vi "_Configure Window.vi"(4 "For Printing (T)":bool=TRUE, 6 "Expt#":i32=1, 7 "ControlRef":T1) -> ()   [LabVIEW 2012]
uses:
  Type/_Run Module.ctl
  Type/_Data Operation.ctl
  Configuration/_Global Configuration.vi
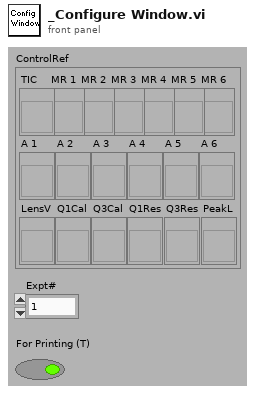
[diagram p1: front panel]
types:
  T1 = cluster{"TIC":refnum<vi>, "MR 1":refnum<vi>, "MR 2":refnum<vi>, "MR 3":refnum<vi>, "MR 4":refnum<vi>, "MR 5":refnum<vi>, "MR 6":refnum<vi>, "A 1":refnum<vi>, "A 2":refnum<vi>, "A 3":refnum<vi>, "A 4":refnum<vi>, "A 5":refnum<vi>, "A 6":refnum<vi>, "LensV":refnum<vi>, "Q1Cal":refnum<vi>, "Q3Cal":refnum<vi>, "Q1Res":refnum<vi>, "Q3Res":refnum<vi>, "PeakL":refnum<vi>}
  T2 = typedef "_Run Module.ctl" = u16
  T3 = typedef "_Data Operation.ctl" = enum8{"Initialize", "Get Data", "Set Data", "Close"}
  T4 = typedef "_Lens Property.ctl" = cluster{"Scan Type":u8, "Scans":i32, "Time 1":dbl, "Time 2":dbl, "Value 1":dbl, "Value 2":dbl, "Step Size":dbl}
  T5 = typedef "_Mass Range Property.ctl" = cluster{"Start":dbl, "Stop":dbl, "Step Size":dbl, "Steps":i32, "Dwell":dbl, "Parameters":T6[], "Res":T7}
  T6 = typedef "_Mass Range Parameters.ctl" = cluster{"Name":string, "Ch#":u8, "StartV":dbl, "StopV":dbl, "StepV":dbl, "Index":u8}
  T7 = typedef "_RT Res Type.ctl" = u16
  T8 = typedef "_Run Mode.ctl" = enum16{"MRM (Q1/Q2)", "Q1 Scan", "Q1 SRM", "Q2 Scan", "Q2 SRM", "Product Scan", "Precursor Scan", "Neutral Loss", "Neutral Gain"}
  T9 = cluster{"Lenses":T4[], "Mass Ranges":T5[], "Acquire":bool, "MCA":bool, "Q1DC EN":bool, "Q1 POL":bool, "Q3 POL":bool, "Q1 RF  EN":bool, "Averaging":bool, "Log Scale":bool, "CPS":bool, "Unit":bool, "Data Path":path, "Run Mode":T8, "Fixed Mass (amu)":dbl, "Q3DC EN":bool, "Q3 RF  EN":bool, "Negative":bool}
  T10 = typedef "_Current Data.ctl" = cluster{"Scan#":i32, "Run Time (mS)":i32, "TIC X":dbl[], "TIC Y":dbl[][], "MassRange":cluster{"X Title":string, "X":dbl[], "Y":i32[]}[], "Fixed Mass (amu)":dbl, "Method":T11}
  T11 = typedef "_XML Expt.ctl" = cluster{"StartT(mS)":i32, "#Cycles":i32, "PauseT(uS)":i32, "ScanType":i32, "Polarity":u8, "FixedMass":dbl, "DelayT(mS)":i32, "Active Ch":T12[], "Mass Range":T5[]}
  T12 = typedef "_XML Lens.ctl" = cluster{"Value":dbl, "ChID":u8}
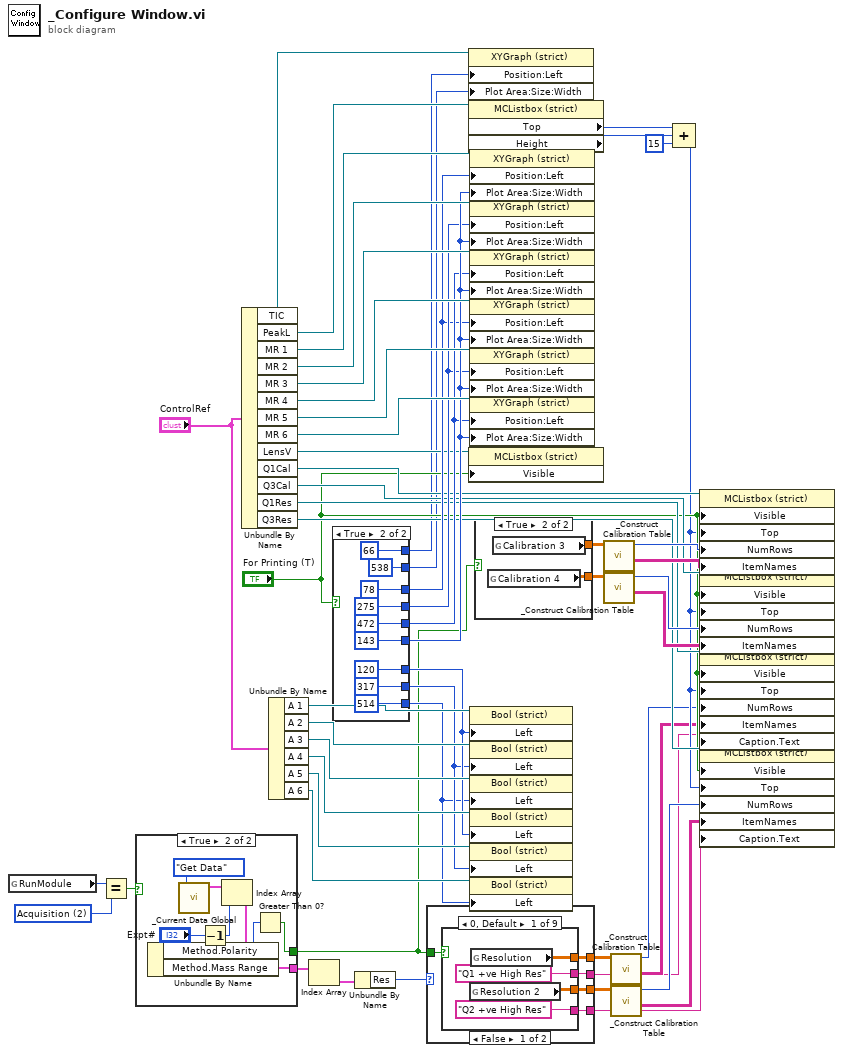
[diagram p0: block diagram]
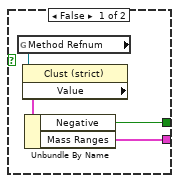
[diagram p2: hidden frame]
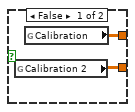
[diagram p3: hidden frame]
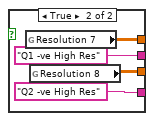
[diagram p4: hidden frame]
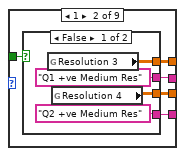
[diagram p5: hidden frame]
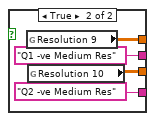
[diagram p6: hidden frame]
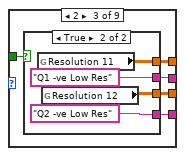
[diagram p7: hidden frame]
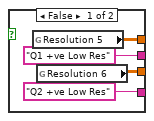
[diagram p8: hidden frame]
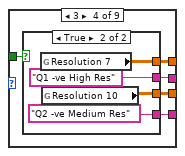
[diagram p9: hidden frame]
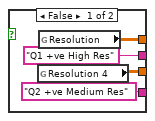
[diagram p10: hidden frame]
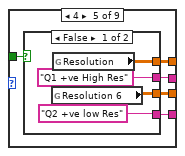
[diagram p11: hidden frame]
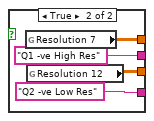
[diagram p12: hidden frame]
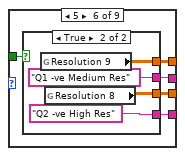
[diagram p13: hidden frame]
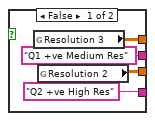
[diagram p14: hidden frame]
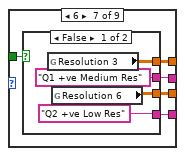
[diagram p15: hidden frame]
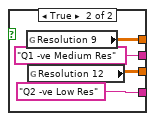
[diagram p16: hidden frame]
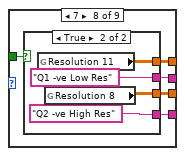
[diagram p17: hidden frame]
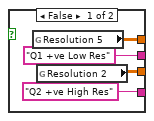
[diagram p18: hidden frame]
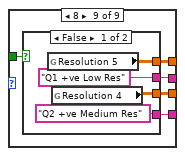
[diagram p19: hidden frame]
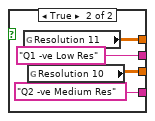
[diagram p20: hidden frame]
diagram:
  w6 = T2 2 items=["Diagnostics", "Tune", "Acquisition"] ("y")
  n1 = global read "_Global Configuration.vi" "RunModule"() -> (w7:T2)
  n2 = Equal?(x=w7, y=w6) -> (x = y?=w5:bool)
  n3 = case shown="True" w5 {
    tunnel: [w57 w63] -> w15
    tunnel: [w56 w62] -> w8
    frame False {
      n4 = global read "_Global Configuration.vi" "Method Refnum"() -> (w59:refnum<vi>)
      n5 = property class="Clust (strict)"(reference=w59) -> ("Value"=w58:T9)  [unwired: 1 in, 2 out]
      n6 = Unbundle By Name(w58) -> ("Negative"=w56:bool, "Mass Ranges"=w57:T5[])
    }
    frame True {
      n7 = call "_Current Data Global.vi"("Operation"=_Data_Operation."Get Data") -> ("CurrentData"=w66:T10[])  [unwired: 3 in, 3 out]
      n8 = Decrement(x="Expt#") -> (x-1=w60:i32)
      n9 = Index Array(array=w66, index=w60) -> (element=w64:T10)
      n10 = Unbundle By Name(w64) -> ("Method.Polarity"=w61:u8, "Method.Mass Range"=w63:T5[])
      n11 = Greater Than 0?(x=w61) -> (x > 0?=w62:bool)
    }
  }
  n12 = Unbundle By Name("ControlRef") -> ("TIC"=w3:refnum<vi>, "PeakL"=w35:refnum<vi>, "MR 1"=w55:refnum<vi>, "MR 2"=w53:refnum<vi>, "MR 3"=w52:refnum<vi>, "MR 4"=w51:refnum<vi>, "MR 5"=w50:refnum<vi>, "MR 6"=w54:refnum<vi>, "LensV"=w45:refnum<vi>, "Q1Cal"=w34:refnum<vi>, "Q3Cal"=w27:refnum<vi>, "Q1Res"=w23:refnum<vi>, "Q3Res"=w22:refnum<vi>)
  n13 = Unbundle By Name("ControlRef") -> ("A 1"=w44:refnum<vi>, "A 2"=w43:refnum<vi>, "A 3"=w42:refnum<vi>, "A 4"=w41:refnum<vi>, "A 5"=w40:refnum<vi>, "A 6"=w39:refnum<vi>)
  n14 = Index Array(array=w15) -> (element=w14:T5)  [unwired: 1 in]
  n15 = case shown="True" "For Printing (T)" {
    tunnel: [-52 ("Position:Left") 78 ("Position:Left")] -> w46
    tunnel: [189 ("Plot Area:Size:Width") 275 ("Plot Area:Size:Width")] -> w47
    tunnel: [429 ("Plot Area:Size:Width") 472 ("Plot Area:Size:Width")] -> w48
    tunnel: [u32 186 ("Plot Area:Size:Width") u32 143 ("Plot Area:Size:Width")] -> w49
    tunnel: [-10 ("Position:Left") 120 ("Position:Left")] -> w38
    tunnel: [231 ("Plot Area:Size:Width") 317 ("Plot Area:Size:Width")] -> w37
    tunnel: [471 ("Plot Area:Size:Width") 514 ("Plot Area:Size:Width")] -> w36
    tunnel: [-64 ("Position:Left") 66 ("Position:Left")] -> w2
    tunnel: [u32 668 ("Plot Area:Size:Width") u32 538 ("Plot Area:Size:Width")] -> w1
    frame False {
    }
    frame True {
    }
  }
  n16 = Unbundle By Name(w14) -> ("Res"=w13:T7)
  n17 = case shown="0, Default" w13 {
    tunnel: [w90 w103 w116 w129 w142 w155 w168 w181 w194] -> w12
    tunnel: [w89 w102 w115 w128 w141 w154 w167 w180 w193] -> w11
    tunnel: [w88 w101 w114 w127 w140 w153 w166 w179 w192] -> w10
    tunnel: [w87 w100 w113 w126 w139 w152 w165 w178 w191] -> w9
    tunnel: w8 -> [w86 w99 w112 w125 w138 w151 w164 w177 w190]
    frame 0, Default {
      n18 = case shown="False" w86 {
        tunnel: [w94 w98] -> w90
        tunnel: [w93 w96] -> w89
        tunnel: ["Q1 +ve High Res" "Q1 -ve High Res"] -> w88
        tunnel: ["Q2 +ve High Res" "Q2 -ve High Res"] -> w87
        frame False {
          n19 = global read "_Global Configuration.vi" "Resolution 2"() -> (w93:dbl[][])
          n20 = global read "_Global Configuration.vi" "Resolution"() -> (w94:dbl[][])
        }
        frame True {
          n21 = global read "_Global Configuration.vi" "Resolution 7"() -> (w98:dbl[][])
          n22 = global read "_Global Configuration.vi" "Resolution 8"() -> (w96:dbl[][])
        }
      }
    }
    frame 1 {
      n23 = case shown="False" w99 {
        tunnel: [w107 w111] -> w103
        tunnel: [w106 w109] -> w102
        tunnel: ["Q1 +ve Medium Res" "Q1 -ve Medium Res"] -> w101
        tunnel: ["Q2 +ve Medium Res" "Q2 -ve Medium Res"] -> w100
        frame False {
          n24 = global read "_Global Configuration.vi" "Resolution 3"() -> (w107:dbl[][])
          n25 = global read "_Global Configuration.vi" "Resolution 4"() -> (w106:dbl[][])
        }
        frame True {
          n26 = global read "_Global Configuration.vi" "Resolution 9"() -> (w111:dbl[][])
          n27 = global read "_Global Configuration.vi" "Resolution 10"() -> (w109:dbl[][])
        }
      }
    }
    frame 2 {
      n28 = case shown="True" w112 {
        tunnel: [w120 w124] -> w116
        tunnel: [w119 w122] -> w115
        tunnel: ["Q1 +ve Low Res" "Q1 -ve Low Res"] -> w114
        tunnel: ["Q2 +ve Low Res" "Q2 -ve Low Res"] -> w113
        frame False {
          n29 = global read "_Global Configuration.vi" "Resolution 5"() -> (w120:dbl[][])
          n30 = global read "_Global Configuration.vi" "Resolution 6"() -> (w119:dbl[][])
        }
        frame True {
          n31 = global read "_Global Configuration.vi" "Resolution 11"() -> (w124:dbl[][])
          n32 = global read "_Global Configuration.vi" "Resolution 12"() -> (w122:dbl[][])
        }
      }
    }
    frame 3 {
      n33 = case shown="True" w125 {
        tunnel: [w133 w137] -> w129
        tunnel: [w132 w135] -> w128
        tunnel: ["Q1 +ve High Res" "Q1 -ve High Res"] -> w127
        tunnel: ["Q2 +ve Medium Res" "Q2 -ve Medium Res"] -> w126
        frame False {
          n34 = global read "_Global Configuration.vi" "Resolution 4"() -> (w132:dbl[][])
          n35 = global read "_Global Configuration.vi" "Resolution"() -> (w133:dbl[][])
        }
        frame True {
          n36 = global read "_Global Configuration.vi" "Resolution 7"() -> (w137:dbl[][])
          n37 = global read "_Global Configuration.vi" "Resolution 10"() -> (w135:dbl[][])
        }
      }
    }
    frame 4 {
      n38 = case shown="False" w138 {
        tunnel: [w146 w150] -> w142
        tunnel: [w145 w148] -> w141
        tunnel: ["Q1 +ve High Res" "Q1 -ve High Res"] -> w140
        tunnel: ["Q2 +ve low Res" "Q2 -ve Low Res"] -> w139
        frame False {
          n39 = global read "_Global Configuration.vi" "Resolution 6"() -> (w145:dbl[][])
          n40 = global read "_Global Configuration.vi" "Resolution"() -> (w146:dbl[][])
        }
        frame True {
          n41 = global read "_Global Configuration.vi" "Resolution 7"() -> (w150:dbl[][])
          n42 = global read "_Global Configuration.vi" "Resolution 12"() -> (w148:dbl[][])
        }
      }
    }
    frame 5 {
      n43 = case shown="True" w151 {
        tunnel: [w159 w163] -> w155
        tunnel: [w158 w161] -> w154
        tunnel: ["Q1 +ve Medium Res" "Q1 -ve Medium Res"] -> w153
        tunnel: ["Q2 +ve High Res" "Q2 -ve High Res"] -> w152
        frame False {
          n44 = global read "_Global Configuration.vi" "Resolution 3"() -> (w159:dbl[][])
          n45 = global read "_Global Configuration.vi" "Resolution 2"() -> (w158:dbl[][])
        }
        frame True {
          n46 = global read "_Global Configuration.vi" "Resolution 9"() -> (w163:dbl[][])
          n47 = global read "_Global Configuration.vi" "Resolution 8"() -> (w161:dbl[][])
        }
      }
    }
    frame 6 {
      n48 = case shown="False" w164 {
        tunnel: [w172 w176] -> w168
        tunnel: [w171 w174] -> w167
        tunnel: ["Q1 +ve Medium Res" "Q1 -ve Medium Res"] -> w166
        tunnel: ["Q2 +ve Low Res" "Q2 -ve Low Res"] -> w165
        frame False {
          n49 = global read "_Global Configuration.vi" "Resolution 3"() -> (w172:dbl[][])
          n50 = global read "_Global Configuration.vi" "Resolution 6"() -> (w171:dbl[][])
        }
        frame True {
          n51 = global read "_Global Configuration.vi" "Resolution 9"() -> (w176:dbl[][])
          n52 = global read "_Global Configuration.vi" "Resolution 12"() -> (w174:dbl[][])
        }
      }
    }
    frame 7 {
      n53 = case shown="True" w177 {
        tunnel: [w185 w189] -> w181
        tunnel: [w184 w187] -> w180
        tunnel: ["Q1 +ve Low Res" "Q1 -ve Low Res"] -> w179
        tunnel: ["Q2 +ve High Res" "Q2 -ve High Res"] -> w178
        frame False {
          n54 = global read "_Global Configuration.vi" "Resolution 5"() -> (w185:dbl[][])
          n55 = global read "_Global Configuration.vi" "Resolution 2"() -> (w184:dbl[][])
        }
        frame True {
          n56 = global read "_Global Configuration.vi" "Resolution 11"() -> (w189:dbl[][])
          n57 = global read "_Global Configuration.vi" "Resolution 8"() -> (w187:dbl[][])
        }
      }
    }
    frame 8 {
      n58 = case shown="False" w190 {
        tunnel: [w198 w202] -> w194
        tunnel: [w197 w200] -> w193
        tunnel: ["Q1 +ve Low Res" "Q1 -ve Low Res"] -> w192
        tunnel: ["Q2 +ve Medium Res" "Q2 -ve Medium Res"] -> w191
        frame False {
          n59 = global read "_Global Configuration.vi" "Resolution 5"() -> (w198:dbl[][])
          n60 = global read "_Global Configuration.vi" "Resolution 4"() -> (w197:dbl[][])
        }
        frame True {
          n61 = global read "_Global Configuration.vi" "Resolution 11"() -> (w202:dbl[][])
          n62 = global read "_Global Configuration.vi" "Resolution 10"() -> (w200:dbl[][])
        }
      }
    }
  }
  n63 = property class="XYGraph (strict)"(reference=w3, "Position:Left"=w2, "Plot Area:Size:Width"=w1) -> ()  [unwired: 1 in, 2 out]
  n64 = property class="MCListbox (strict)"(reference=w35) -> ("Top"=w33:i32, "Height"=w32:u32)  [unwired: 1 in, 2 out]
  n65 = property class="MCListbox (strict)"(reference=w45, "Visible"="For Printing (T)") -> ()  [unwired: 1 in, 2 out]
  n66 = property class="XYGraph (strict)"(reference=w55, "Position:Left"=w46, "Plot Area:Size:Width"=w49) -> ()  [unwired: 1 in, 2 out]
  n67 = property class="XYGraph (strict)"(reference=w53, "Position:Left"=w47, "Plot Area:Size:Width"=w49) -> ()  [unwired: 1 in, 2 out]
  n68 = property class="XYGraph (strict)"(reference=w52, "Position:Left"=w48, "Plot Area:Size:Width"=w49) -> ()  [unwired: 1 in, 2 out]
  n69 = property class="XYGraph (strict)"(reference=w51, "Position:Left"=w46, "Plot Area:Size:Width"=w49) -> ()  [unwired: 1 in, 2 out]
  n70 = property class="XYGraph (strict)"(reference=w50, "Position:Left"=w47, "Plot Area:Size:Width"=w49) -> ()  [unwired: 1 in, 2 out]
  n71 = property class="XYGraph (strict)"(reference=w54, "Position:Left"=w48, "Plot Area:Size:Width"=w49) -> ()  [unwired: 1 in, 2 out]
  n72 = property class="Bool (strict)"(reference=w44, "Left"=w38) -> ()  [unwired: 1 in, 2 out]
  n73 = property class="Bool (strict)"(reference=w43, "Left"=w37) -> ()  [unwired: 1 in, 2 out]
  n74 = property class="Bool (strict)"(reference=w42, "Left"=w36) -> ()  [unwired: 1 in, 2 out]
  n75 = property class="Bool (strict)"(reference=w41, "Left"=w38) -> ()  [unwired: 1 in, 2 out]
  n76 = property class="Bool (strict)"(reference=w40, "Left"=w37) -> ()  [unwired: 1 in, 2 out]
  n77 = property class="Bool (strict)"(reference=w39, "Left"=w36) -> ()  [unwired: 1 in, 2 out]
  n78 = case shown="True" w8 {
    tunnel: [w204 w206] -> w30
    tunnel: [w203 w205] -> w26
    frame False {
      n79 = global read "_Global Configuration.vi" "Calibration 2"() -> (w203:dbl[][])
      n80 = global read "_Global Configuration.vi" "Calibration"() -> (w204:dbl[][])
    }
    frame True {
      n81 = global read "_Global Configuration.vi" "Calibration 4"() -> (w205:dbl[][])
      n82 = global read "_Global Configuration.vi" "Calibration 3"() -> (w206:dbl[][])
    }
  }
  n83 = call "_Construct Calibration Table.vi"("Calibration"=w30) -> ("Table"=w28:string[][], "Rows"=w29:i32)  [unwired: 5 out]
  n84 = call "_Construct Calibration Table.vi"("Calibration"=w26) -> ("Table"=w24:string[][], "Rows"=w25:i32)  [unwired: 5 out]
  n85 = call "_Construct Calibration Table.vi"("Calibration"=w12) -> ("Table"=w18:string[][], "Rows"=w19:i32)  [unwired: 5 out]
  n86 = call "_Construct Calibration Table.vi"("Calibration"=w11) -> ("Table"=w16:string[][], "Rows"=w17:i32)  [unwired: 5 out]
  n87 = Compound Arithmetic op=ADD(w33, w32, u32 15 ("value")) -> (w20:u32)
  n88 = property class="MCListbox (strict)"(reference=w34, "Visible"="For Printing (T)", "Top"=w20, "NumRows"=w29, "ItemNames"=w28) -> ()  [unwired: 1 in, 2 out]
  n89 = property class="MCListbox (strict)"(reference=w27, "Visible"="For Printing (T)", "Top"=w20, "NumRows"=w25, "ItemNames"=w24) -> ()  [unwired: 1 in, 2 out]
  n90 = property class="MCListbox (strict)"(reference=w23, "Visible"="For Printing (T)", "Top"=w20, "NumRows"=w19, "ItemNames"=w18, "Caption.Text"=w10) -> ()  [unwired: 1 in, 2 out]
  n91 = property class="MCListbox (strict)"(reference=w22, "Visible"="For Printing (T)", "Top"=w20, "NumRows"=w17, "ItemNames"=w16, "Caption.Text"=w9) -> ()  [unwired: 1 in, 2 out]
